vi "json Insert String - array path.vi"(8 "error in (no error)":errorcluster, 9 "anything":string, 10 "path":string[](array[string]), 11 "JSON Document in":refnum<class "JSON Document.lvclass">) -> (0 "error out":errorcluster, 3 "JSON Document out":refnum<class "JSON Document.lvclass">)   [LabVIEW 2015, in "JSON Document.lvclass"]
uses:
  JSON Document.lvclass
  json Insert String - string path.vi
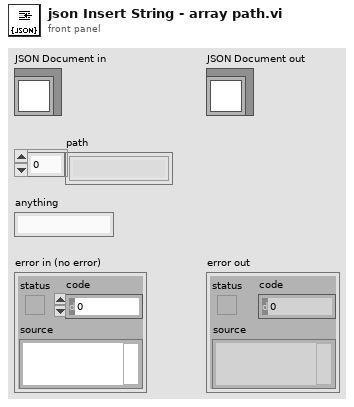
[diagram p1: front panel]
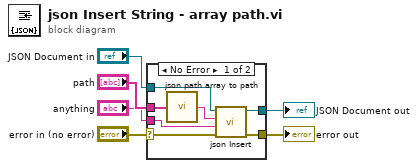
[diagram p0: block diagram]
diagram:
  n1 = case shown="No Error" "error in (no error)" {
    selector: "error in (no error)" -> [w9 w15]
    tunnel: [w10 w15] -> w2
    tunnel: [w11 w14] -> w1
    tunnel: "JSON Document in" -> [w12 w14]
    tunnel: "anything" -> [w8 _]
    tunnel: "path" -> [w7 _]
    frame No Error {
      n2 = call "json path array to path.vi"("path"=w7) -> ("String"=w13:string)
      n3 = call-poly "json Insert.vi"("error in (no error)"=w9, "anything"=w8, "path"=w13, "JSON Document in"=w12) -> ("error out"=w10:errorcluster, "JSON Document out"=w11:refnum<class "JSON Document.lvclass">)  [unwired: 6 in]
    }
    frame Error {
    }
  }
  "error out" <- w2
  "JSON Document out" <- w1
